vi "ex8.vi"() -> ()   [LabVIEW 2022 SP3]
uses:
  <vilib>/numeric/Random Number (Range) DBL.vi
panel:
  out "concatenated string":string
  in  "stop":bool
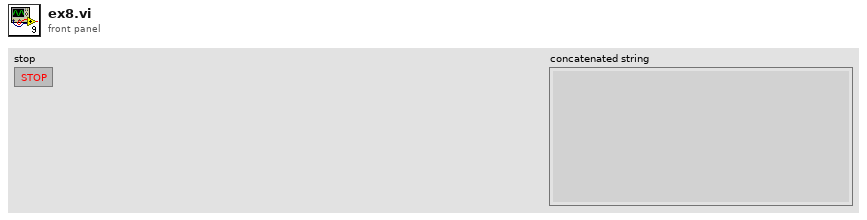
[diagram p1: front panel]
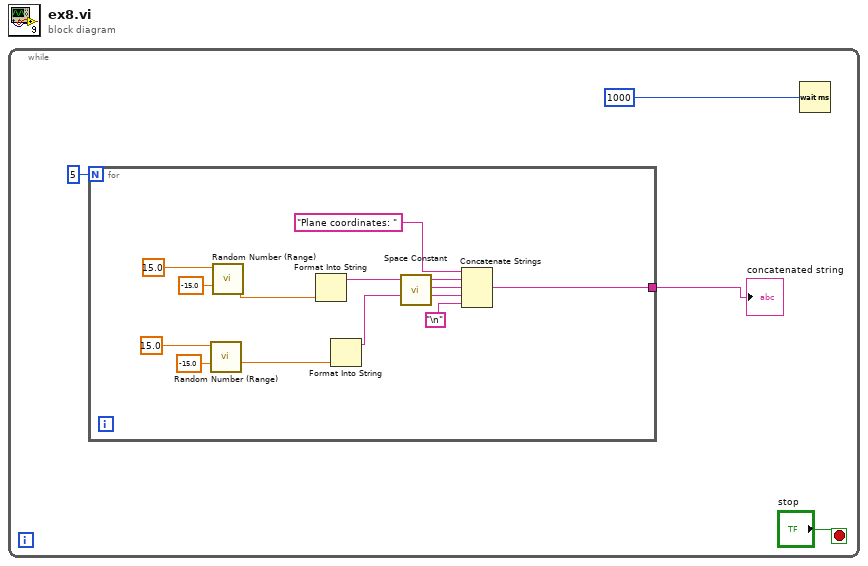
[diagram p0: block diagram]
diagram:
  n1 = while {
    stop <- "stop" stop-if-true
    n2 = for {
      N: 5 -> [_]
      tunnel: [w5] -> w1
      n3 = call-poly <vilib>:"Random Number (Range).vi"("lower bound (0)"=-15.0, "upper bound (100)"=15.0) -> ("number"=w9:dbl)  [unwired: 9 in]
      n4 = call-poly <vilib>:"Random Number (Range).vi"("lower bound (0)"=-15.0, "upper bound (100)"=15.0) -> ("number"=w10:dbl)  [unwired: 9 in]
      n5 = Format Into String(w10) -> (resulting string=w8:string)  [unwired: 3 in, 1 out]
      n6 = Format Into String(w9) -> (resulting string=w7:string)  [unwired: 3 in, 1 out]
      n7 = call <vilib>:"Space Constant.vi"() -> ("String"=w11:string)
      n8 = Concatenate Strings("Plane coordinates: " ("string"), w8, w11, w7, "\n") -> (w5:string)
    }
    "concatenated string" <- w1
    n9 = Wait (ms)(milliseconds to wait=u32 1000) -> ()  [unwired: 1 out]
  }
